vi "Config Read Sequence Steps.vi"(8 "Error In":errorcluster, 9 "Base Path":path=path "C:/Labview Code/System/Part Configuration", 11 "Station Name":string) -> (0 "Error Out":errorcluster, 2 "VI Names":string[](array[string]), 3 "Sequence Steps":string[](array[string]))   [LabVIEW 2018]
uses:
  <vilib>/Utility/config.llb/Read Key (String).vi
  <vilib>/Utility/config.llb/NI_LVConfig.lvlib
panel:
  out "All Keys":string[](array[string])
  out "All Sections":string[](array[string])
  # "6"
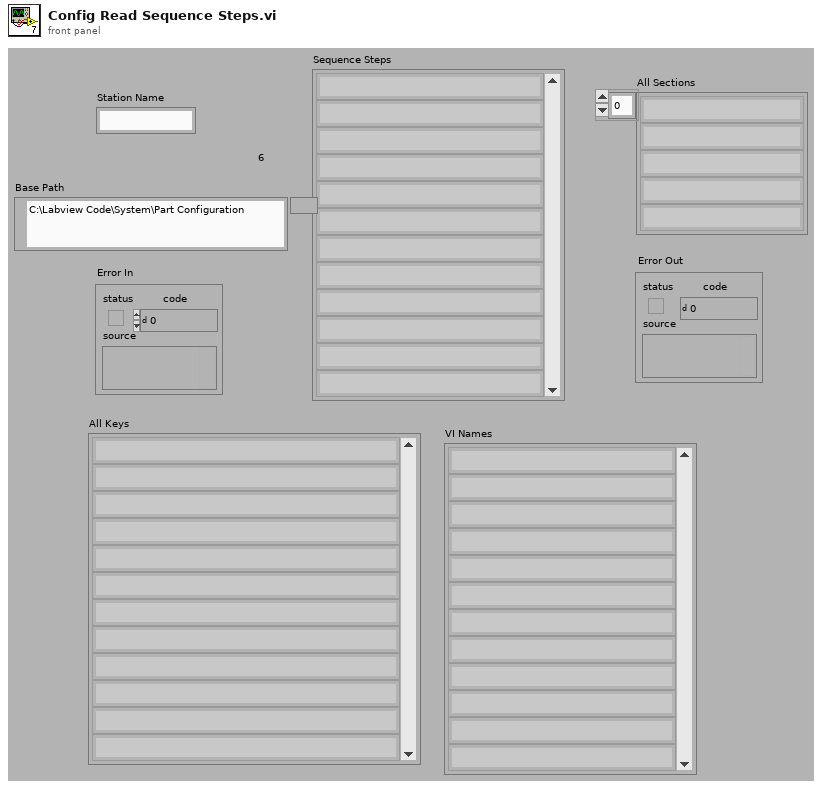
[diagram p1: front panel]
types:
  T1 = typedef "NI_LVConfig.lvlib/Config Data RefNum.ctl" = refnum<k1>
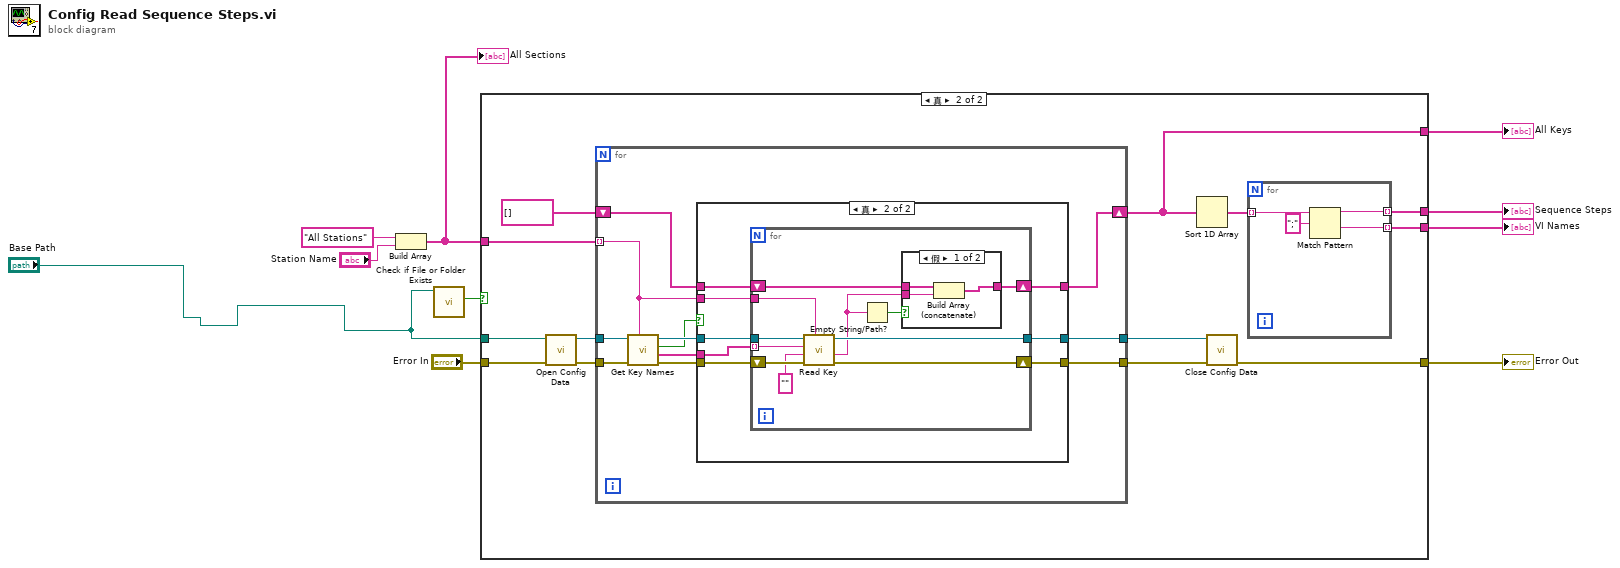
[diagram p0: block diagram]
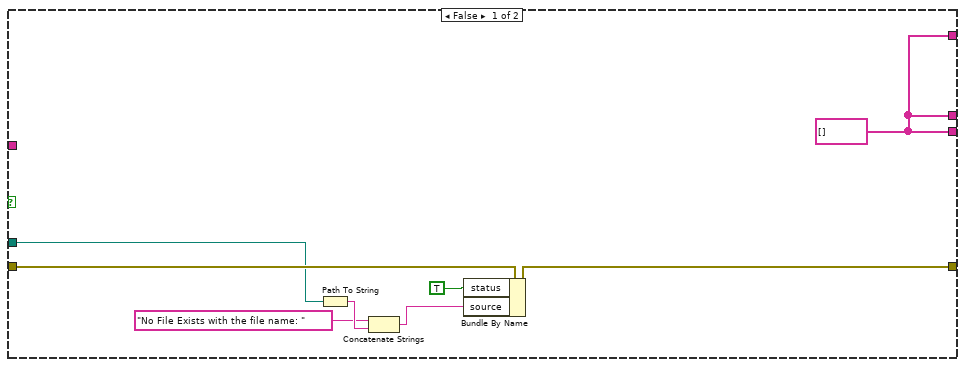
[diagram p2: hidden frame]
diagram:
  n1 = Build Array("All Stations", "Station Name") -> (w6:string[])
  "All Sections" <- w6
  n2 = call <vilib>:"Check if File or Folder Exists.vi"("path"="Base Path") -> ("file or folder exists?"=w5:bool)  [unwired: 8 in, 2 out]
  n3 = case shown="真" w5 {
    tunnel: "Base Path" -> [w12 w31]
    tunnel: [w16 w26] -> w10
    tunnel: "Error In" -> [w17 w25]
    tunnel: [w11 w24] -> w2
    tunnel: [w11 w23] -> w1
    tunnel: [w11 w21] -> w8
    tunnel: w6 -> [_ w20]
    frame False {
      w11 = string[] []
      n4 = Path To String(path=w12) -> (string=w15:string)
      n5 = Concatenate Strings("No File Exists with the file name: " ("string"), w15) -> (w13:string)
      n6 = Bundle By Name(cluster=w17, "status"=TRUE, "source"=w13) -> (w16:errorcluster)
    }
    frame True {
      n7 = call <vilib>:"Open Config Data.vi"("error in (no error)"=w25, "configuration file path"=w31) -> ("error out"=w29:errorcluster, "refnum"=w30:T1)  [unwired: 7 in, 1 out]
      n8 = for {
        tunnel: w30 -> [w46]
        tunnel: w29 -> [w45]
        tunnel: [w41] -> w28
        tunnel: [w40] -> w27
        tunnel: w20 -> [w39] mode=indexing
        shift-right: [w37] -> w21
        shift-left: string[] [] -> [w38]
        n9 = call <vilib>:"Get Key Names.vi"("section"=w39, "error in (no error)"=w45, "refnum"=w46) -> ("error out"=w44:errorcluster, "key names"=w36:string[], "section exists?"=w42:bool, "refnum out"=w43:T1)  [unwired: 5 in]
        n10 = case shown="真" w42 {
          tunnel: w36 -> [_ w57]
          tunnel: w44 -> [w49 w56]
          tunnel: w43 -> [w48 w55]
          tunnel: w39 -> [_ w54]
          tunnel: [w49 w53] -> w41
          tunnel: [w47 w52] -> w37
          tunnel: [w48 w51] -> w40
          tunnel: w38 -> [w47 w50]
          frame False {
          }
          frame True {
            n11 = for {
              tunnel: w57 -> [w66] mode=indexing
              tunnel: w55 -> [w68]
              tunnel: w54 -> [w67]
              shift-right: [w64] -> w53
              shift-left: w56 -> [w65]
              tunnel: [w62] -> w51
              shift-right: [w61] -> w52
              shift-left: w50 -> [w60]
              n12 = call-poly <vilib>:"Read Key.vi"("section"=w67, "error in (no error)"=w65, "default value"="", "key"=w66, "refnum"=w68) -> ("error out"=w64:errorcluster, "value"=w58:string, "refnum out"=w62:T1)  [unwired: 3 in, 1 out]
              n13 = Empty String/Path?(string/path=w58) -> (empty?=w59:bool)
              n14 = case shown="假" w59 {
                tunnel: w58 -> [w71 _]
                tunnel: [w70 w72] -> w61
                tunnel: w60 -> [w69 w72]
                frame False {
                  n15 = Build Array (concatenate)(w69, w71) -> (w70:string[])
                }
                frame True {
                }
              }
            }
          }
        }
      }
      n16 = Sort 1D Array(array=w21) -> (sorted array=w22:string[])
      n17 = call <vilib>:"Close Config Data.vi"("error in (no error)"=w28, "refnum"=w27) -> ("error out"=w26:errorcluster)  [unwired: 8 in, 1 out]
      n18 = for {
        tunnel: w22 -> [w35] mode=indexing
        tunnel: [w34] -> w23 mode=indexing
        tunnel: [w32] -> w24 mode=indexing
        n19 = Match Pattern(string=w35, regular expression=";") -> (before substring=w34:string, after substring=w32:string)  [unwired: 1 in, 2 out]
      }
    }
  }
  "Sequence Steps" <- w1
  "Error Out" <- w10
  "VI Names" <- w2
  "All Keys" <- w8
